vi "CharToBoolean(cast).vi"(1 "Str":string) -> (0 "Boolean":bool)   [LabVIEW 2012]
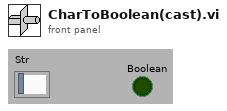
[diagram p1: front panel]
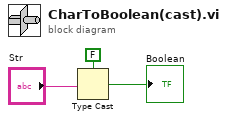
[diagram p0: block diagram]
diagram:
  n1 = Type Cast(type=FALSE ("Boolean"), x="Str") -> (*(type *) &x=→"Boolean":bool)
